vi "WT210 Element Data.vi"(4 "Uthd:Element 2":dbl, 5 "C Factor (0: V) 2":u16, 6 "Uthd:Element 1":dbl, 7 "Element (1: Element 1)":u16, 8 "error in (no error)":errorcluster, 9 "C Factor (0: V)":u16, 10 "Dryer PowerData in":T1 {"Voltage (V):Element 1 Avg" format="%.3g"; "Voltage (V):Element 2 Avg" format="%.3g"; "Max Watt Hours" format="%.3g"; "Power Factor:Element 2" format="%.3g"; "Power Factor:Element 1" format="%.3g"; "Apparent Power (VA):Element 2" format="%.3g"; "Apparent Power (VA):Element 1" format="%.3g"; "Frequency (Hz):Element 1" format="%.3g"; "Time:Element 1" format="%.3g"; "Voltage Crest Factor:Element 2" format="%.3g"; "Voltage Crest Factor:Element 1" format="%.3g"; "Voltage Harmonic (%):Element 2" format="%.3g"; "Voltage Harmonic (%):Element 1" format="%.3g"; "Current Crest Factor:Element 2" format="%.3g"; "Current Crest Factor:Element 1" format="%.3g"; "Voltage (V):Element 1" format="%.3g"; "Voltage (V):Element 2" format="%.3g"; "Watt Hours (Wh):Sigma" format="%.3f"; "Power (W):Sigma" format="%.3g"; "Current (A):Element 2" format="%.3g"; "Current (A):Element 1" format="%.3g"}, 11 "VISA Refnum in":refnum<visa-resource-name>) -> (0 "error out":errorcluster, 2 "Dryer PowerData out":T1 {"Voltage (V):Element 1 Avg" format="%.3g"; "Voltage (V):Element 2 Avg" format="%.3g"; "Max Watt Hours" format="%.3g"; "Power Factor:Element 2" format="%.3g"; "Power Factor:Element 1" format="%.3g"; "Apparent Power (VA):Element 2" format="%.3g"; "Apparent Power (VA):Element 1" format="%.3g"; "Frequency (Hz):Element 1" format="%.3g"; "Time:Element 1" format="%.3g"; "Voltage Crest Factor:Element 2" format="%.3g"; "Voltage Crest Factor:Element 1" format="%.3g"; "Voltage Harmonic (%):Element 2" format="%.3g"; "Voltage Harmonic (%):Element 1" format="%.3g"; "Current Crest Factor:Element 2" format="%.3g"; "Current Crest Factor:Element 1" format="%.3g"; "Voltage (V):Element 1" format="%.3g"; "Voltage (V):Element 2" format="%.3g"; "Watt Hours (Wh):Sigma" format="%.3f"; "Power (W):Sigma" format="%.3g"; "Current (A):Element 2" format="%.3g"; "Current (A):Element 1" format="%.3g"}, 3 "VISA Refnum out":refnum<visa-resource-name>)   [LabVIEW 2018]
uses:
  Trunk/Utility/Type Definitions/UTILITY Power Data.ctl
  Yokogawa WT200 Series.lvlib
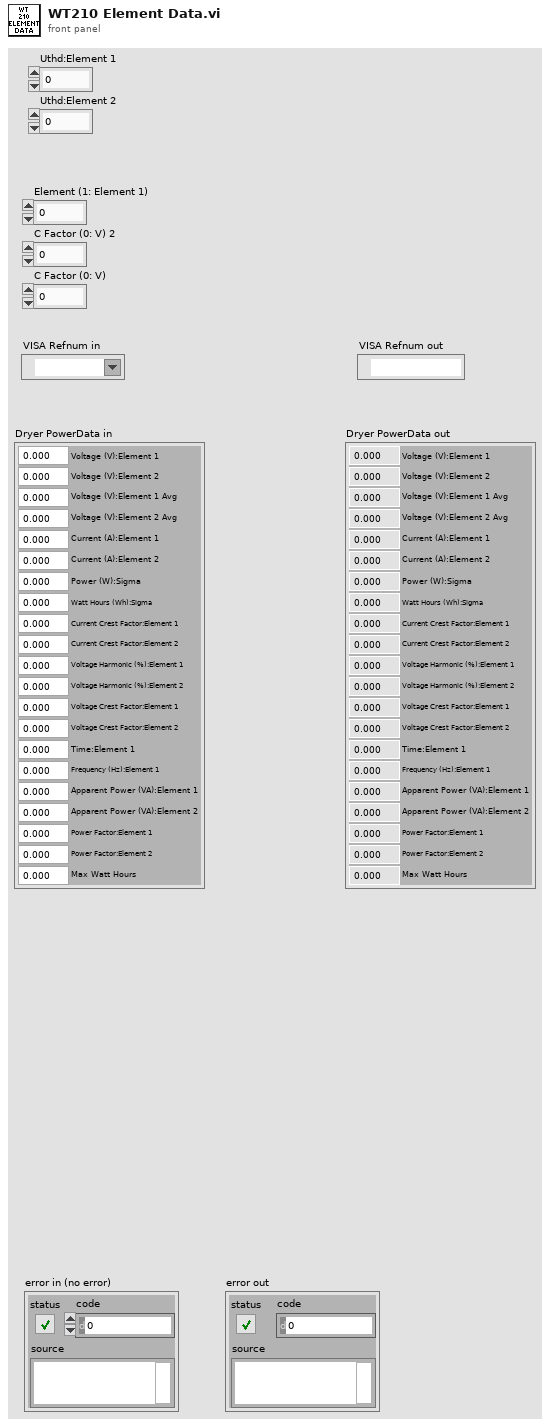
[diagram p1: front panel]
types:
  T1 = typedef "UTILITY Power Data.ctl" = cluster{"Current (A):Element 1":dbl, "Current (A):Element 2":dbl, "Power (W):Sigma":dbl, "Watt Hours (Wh):Sigma":dbl, "Voltage (V):Element 2":dbl, "Voltage (V):Element 1":dbl, "Current Crest Factor:Element 1":dbl, "Current Crest Factor:Element 2":dbl, "Voltage Harmonic (%):Element 1":dbl, "Voltage Harmonic (%):Element 2":dbl, "Voltage Crest Factor:Element 1":dbl, "Voltage Crest Factor:Element 2":dbl, "Time:Element 1":dbl, "Frequency (Hz):Element 1":dbl, "Apparent Power (VA):Element 1":dbl, "Apparent Power (VA):Element 2":dbl, "Power Factor:Element 1":dbl, "Power Factor:Element 2":dbl, "Max Watt Hours":dbl, "Voltage (V):Element 2 Avg":dbl, "Voltage (V):Element 1 Avg":dbl}
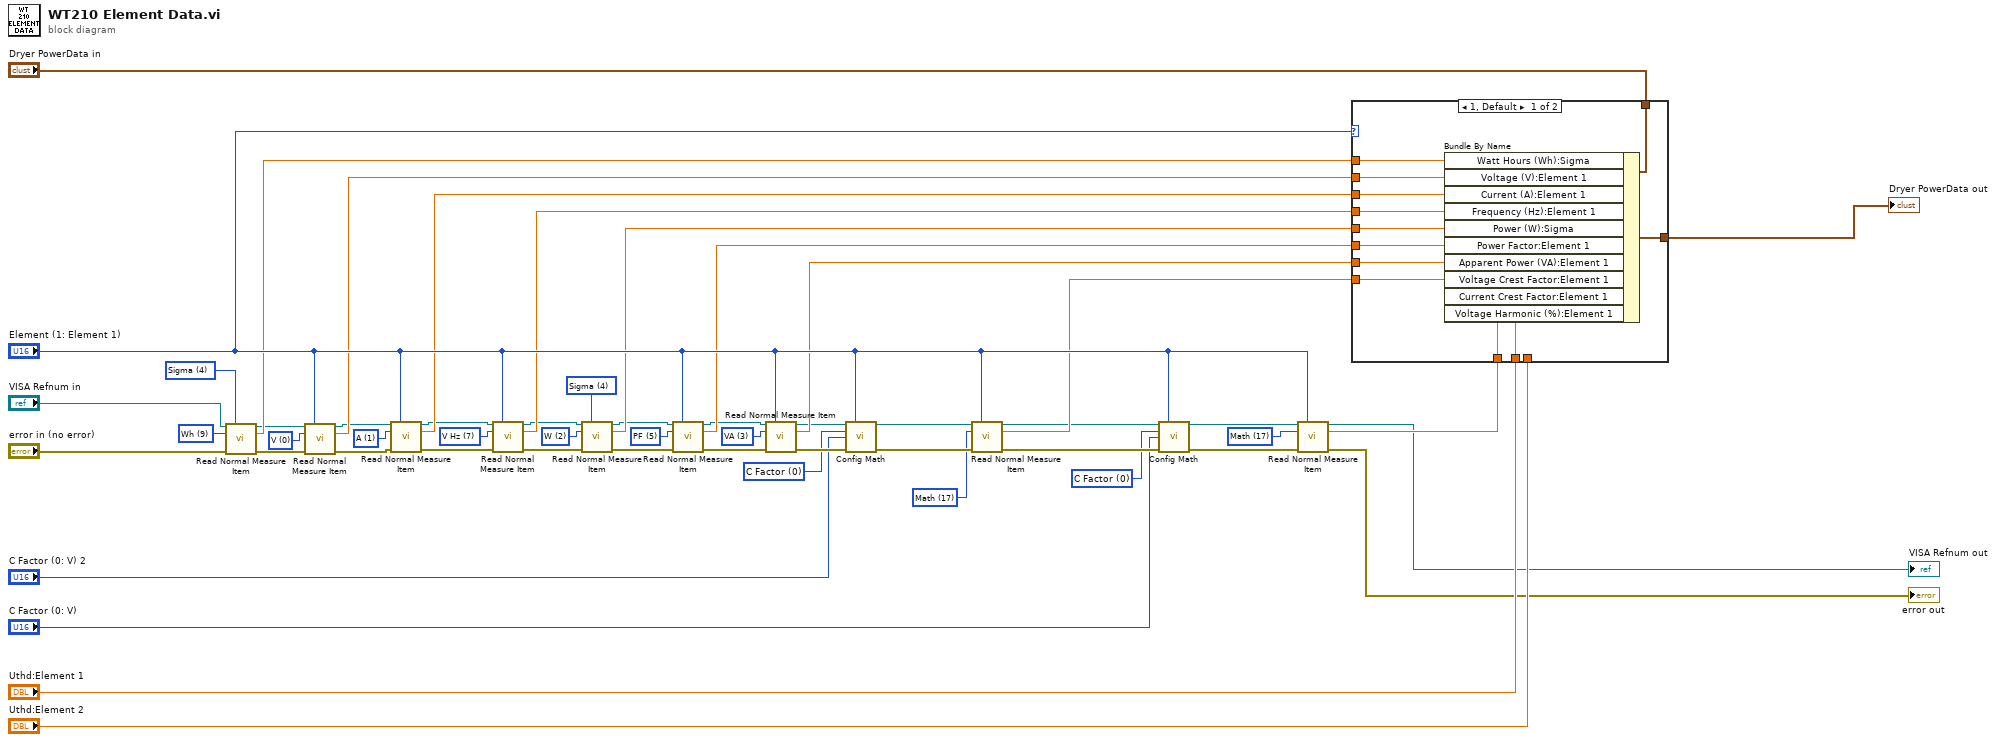
[diagram p0: block diagram]
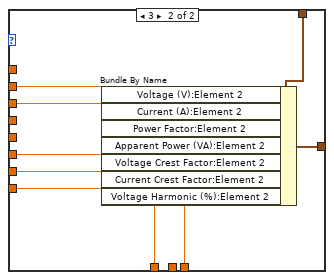
[diagram p2: hidden frame]
diagram:
  w1 = u16 4 items=["", "Element1", "Element2", "Element3", "Sigma"] ("Element (1: Element 1)")
  w2 = u16 4 items=["", "Element1", "Element2", "Element3", "Sigma"] ("Element (1: Element 1)")
  w40 = u16 17 items=["V", "A", "W", "VA", "var", "PF", "deg", "V Hz", "A Hz", "Wh", "Wh+", "Wh-", "Ah", "Ah+", "Ah-", "Vpk", "Apk", "Math"] ("Measure Item (0: V)")
  w35 = u16 0 items=["C Factor", "Arithmetic", "Average", "Efficiency"] ("Math Type (0: Crest Factor)")
  w30 = u16 0 items=["C Factor", "Arithmetic", "Average", "Efficiency"] ("Math Type (0: Crest Factor)")
  w28 = u16 17 items=["V", "A", "W", "VA", "var", "PF", "deg", "V Hz", "A Hz", "Wh", "Wh+", "Wh-", "Ah", "Ah+", "Ah-", "Vpk", "Apk", "Math"] ("Measure Item (0: V)")
  w21 = u16 3 items=["V", "A", "W", "VA", "var", "PF", "deg", "V Hz", "A Hz", "Wh", "Wh+", "Wh-", "Ah", "Ah+", "Ah-", "Vpk", "Apk", "Math"] ("Measure Item (0: V)")
  w20 = u16 5 items=["V", "A", "W", "VA", "var", "PF", "deg", "V Hz", "A Hz", "Wh", "Wh+", "Wh-", "Ah", "Ah+", "Ah-", "Vpk", "Apk", "Math"] ("Measure Item (0: V)")
  w19 = u16 2 items=["V", "A", "W", "VA", "var", "PF", "deg", "V Hz", "A Hz", "Wh", "Wh+", "Wh-", "Ah", "Ah+", "Ah-", "Vpk", "Apk", "Math"] ("Measure Item (0: V)")
  w18 = u16 7 items=["V", "A", "W", "VA", "var", "PF", "deg", "V Hz", "A Hz", "Wh", "Wh+", "Wh-", "Ah", "Ah+", "Ah-", "Vpk", "Apk", "Math"] ("Measure Item (0: V)")
  w17 = u16 1 items=["V", "A", "W", "VA", "var", "PF", "deg", "V Hz", "A Hz", "Wh", "Wh+", "Wh-", "Ah", "Ah+", "Ah-", "Vpk", "Apk", "Math"] ("Measure Item (0: V)")
  w16 = u16 0 items=["V", "A", "W", "VA", "var", "PF", "deg", "V Hz", "A Hz", "Wh", "Wh+", "Wh-", "Ah", "Ah+", "Ah-", "Vpk", "Apk", "Math"] ("Measure Item (0: V)")
  w9 = u16 9 items=["V", "A", "W", "VA", "var", "PF", "deg", "V Hz", "A Hz", "Wh", "Wh+", "Wh-", "Ah", "Ah+", "Ah-", "Vpk", "Apk", "Math"] ("Measure Item (0: V)")
  n1 = call "Read Normal Measure Item.vi"("VISA resource name"="VISA Refnum in", "Element (1: Element 1)"=w2, "Measure Item (0: V)"=w9, "error in (no error)"="error in (no error)") -> ("VISA resource name out"=w15:refnum<visa-resource-name>, "Measure Value"=w51:sgl, "error out"=w12:errorcluster)  [unwired: 9 in]
  n2 = call "Read Normal Measure Item.vi"("VISA resource name"=w15, "Element (1: Element 1)"="Element (1: Element 1)", "Measure Item (0: V)"=w16, "error in (no error)"=w12) -> ("VISA resource name out"=w13:refnum<visa-resource-name>, "Measure Value"=w43:sgl, "error out"=w10:errorcluster)  [unwired: 9 in]
  n3 = call "Read Normal Measure Item.vi"("VISA resource name"=w13, "Element (1: Element 1)"="Element (1: Element 1)", "Measure Item (0: V)"=w17, "error in (no error)"=w10) -> ("VISA resource name out"=w14:refnum<visa-resource-name>, "Measure Value"=w42:sgl, "error out"=w11:errorcluster)  [unwired: 9 in]
  n4 = call "Read Normal Measure Item.vi"("VISA resource name"=w14, "Element (1: Element 1)"="Element (1: Element 1)", "Measure Item (0: V)"=w18, "error in (no error)"=w11) -> ("VISA resource name out"=w27:refnum<visa-resource-name>, "Measure Value"=w45:sgl, "error out"=w24:errorcluster)  [unwired: 9 in]
  n5 = call "Read Normal Measure Item.vi"("VISA resource name"=w27, "Element (1: Element 1)"=w1, "Measure Item (0: V)"=w19, "error in (no error)"=w24) -> ("VISA resource name out"=w25:refnum<visa-resource-name>, "Measure Value"=w46:sgl, "error out"=w22:errorcluster)  [unwired: 9 in]
  n6 = call "Read Normal Measure Item.vi"("VISA resource name"=w25, "Element (1: Element 1)"="Element (1: Element 1)", "Measure Item (0: V)"=w20, "error in (no error)"=w22) -> ("VISA resource name out"=w26:refnum<visa-resource-name>, "Measure Value"=w47:sgl, "error out"=w23:errorcluster)  [unwired: 9 in]
  n7 = call "Read Normal Measure Item.vi"("VISA resource name"=w26, "Element (1: Element 1)"="Element (1: Element 1)", "Measure Item (0: V)"=w21, "error in (no error)"=w23) -> ("VISA resource name out"=w33:refnum<visa-resource-name>, "Measure Value"=w48:sgl, "error out"=w31:errorcluster)  [unwired: 9 in]
  n8 = call "Config Math.vi"("VISA resource name"=w33, "Element (1: Element 1)"="Element (1: Element 1)", "Math Type (0: Crest Factor)"=w30, "C Factor (0: V)"="C Factor (0: V) 2", "error in (no error)"=w31) -> ("VISA resource name out"=w34:refnum<visa-resource-name>, "error out"=w32:errorcluster)  [unwired: 9 in]
  n9 = call "Read Normal Measure Item.vi"("VISA resource name"=w34, "Element (1: Element 1)"="Element (1: Element 1)", "Measure Item (0: V)"=w28, "error in (no error)"=w32) -> ("VISA resource name out"=w41:refnum<visa-resource-name>, "Measure Value"=w49:sgl, "error out"=w37:errorcluster)  [unwired: 9 in]
  n10 = call "Config Math.vi"("VISA resource name"=w41, "Element (1: Element 1)"="Element (1: Element 1)", "Math Type (0: Crest Factor)"=w35, "C Factor (0: V)"="C Factor (0: V)", "error in (no error)"=w37) -> ("VISA resource name out"=w38:refnum<visa-resource-name>, "error out"=w39:errorcluster)  [unwired: 9 in]
  n11 = call "Read Normal Measure Item.vi"("VISA resource name"=w38, "Element (1: Element 1)"="Element (1: Element 1)", "Measure Item (0: V)"=w40, "error in (no error)"=w39) -> ("VISA resource name out"=→"VISA Refnum out":refnum<visa-resource-name>, "Measure Value"=w44:sgl, "error out"=→"error out":errorcluster)  [unwired: 9 in]
  n12 = case shown="1, Default" "Element (1: Element 1)" {
    tunnel: [w65 w73] -> w5
    tunnel: "Dryer PowerData in" -> [w64 w74]
    tunnel: w42 -> [w63 w71]
    tunnel: w43 -> [w62 w72]
    tunnel: w44 -> [w61 w67]
    tunnel: w45 -> [w60 _]
    tunnel: w46 -> [w59 _]
    tunnel: w47 -> [w58 w70]
    tunnel: w48 -> [w57 w69]
    tunnel: w49 -> [w56 w68]
    tunnel: "Uthd:Element 1" -> [w55 _]
    tunnel: w51 -> [w54 _]
    tunnel: "Uthd:Element 2" -> [_ w66]
    frame 1, Default {
      n13 = Bundle By Name(cluster=w64, "Watt Hours (Wh):Sigma"=w54, "Voltage (V):Element 1"=w62, "Current (A):Element 1"=w63, "Frequency (Hz):Element 1"=w60, "Power (W):Sigma"=w59, "Power Factor:Element 1"=w58, "Apparent Power (VA):Element 1"=w57, "Voltage Crest Factor:Element 1"=w56, "Current Crest Factor:Element 1"=w61, "Voltage Harmonic (%):Element 1"=w55) -> (w65:T1)
    }
    frame 3 {
      n14 = Bundle By Name(cluster=w74, "Voltage (V):Element 2"=w72, "Current (A):Element 2"=w71, "Power Factor:Element 2"=w70, "Apparent Power (VA):Element 2"=w69, "Voltage Crest Factor:Element 2"=w68, "Current Crest Factor:Element 2"=w67, "Voltage Harmonic (%):Element 2"=w66) -> (w73:T1)
    }
  }
  "Dryer PowerData out" <- w5
